vi "Open_Instr.vi"(8 "error in (no error)":errorcluster caption="entrée d'erreur (pas d'erreur)", 11 "Class Multimeter Multimeter en entrée":refnum<class "Class Instrument Schielding_Box.lvclass">) -> (0 "error out":errorcluster caption="sortie d'erreur", 3 "Class Multimeter Multimeter en sortie":refnum<class "Class Instrument Schielding_Box.lvclass">)   [LabVIEW 2020, in "Library Instrument & Equipement.lvlib" / "Library Instruments.lvlib" / "Class Instrument Schielding_Box.lvclass"]
uses:
  Class Instrument Schielding_Box.lvclass
  Class Instrument Schielding_Box.lvclass/Class Instrument Schielding_Box.ctl
  Instrument (Default)/Class Instrument (Default).lvclass
  Shielding box/Class Shielding box (Default)/Class Shielding_ Box (Default).lvclass
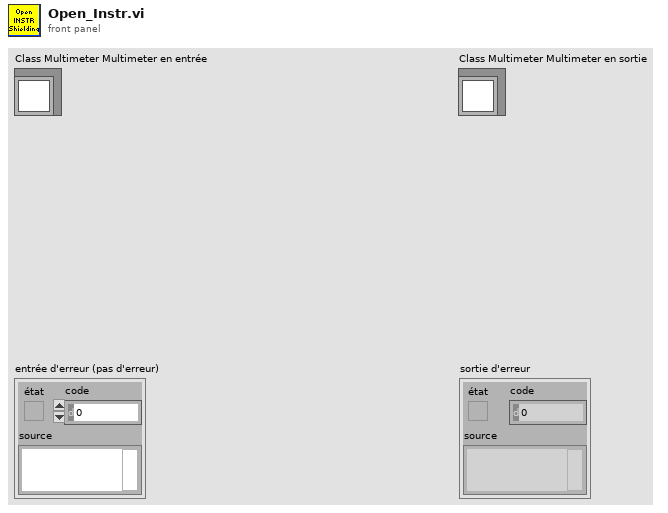
[diagram p1: front panel]
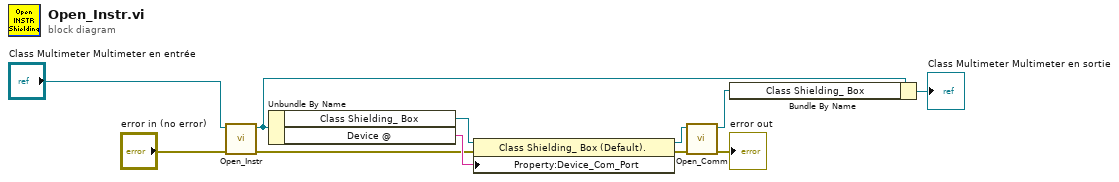
[diagram p0: block diagram]
diagram:
  n1 = call-parent "Open_Instr.vi"("error in (no error)"="error in (no error)", "Class Multimeter (Default) en entrée"="Class Multimeter Multimeter en entrée") -> ("error out"=w5:errorcluster, "Class Multimeter (Default) en sortie"=w8:refnum<class "Class Instrument Schielding_Box.lvclass">)  [unwired: 8 in]
  n2 = Unbundle By Name(w8) -> ("Class Shielding_ Box"=w6:refnum<class "Class Shielding_ Box (Default).lvclass">, "Device @"=w7:string)
  n3 = property class="Class Shielding_ Box (Default)."(reference=w6, error in=w5, "Property:Device_Com_Port"=w7) -> (reference out=w3:refnum<class "Class Shielding_ Box (Default).lvclass">, error out=w4:errorcluster)
  n4 = call-dynamic "Open_Comm.vi"("error in (no error)"=w4, "Class Shielding_ Box en entrée"=w3) -> ("error out"=→"error out":errorcluster, "Class Shielding_ Box en sortie"=w1:refnum<class "Class Shielding_ Box (Default).lvclass">)  [unwired: 8 in]
  n5 = Bundle By Name(cluster=w8, "Class Shielding_ Box"=w1) -> (→"Class Multimeter Multimeter en sortie":refnum<class "Class Instrument Schielding_Box.lvclass">)
